vi "BBoxOne.vi"() -> ()   [LabVIEW 2021]
uses:
  D:/tmytek/Source/bbox-api/example/BBoxOne Series/LabVIEW/BBoxAPI.dll
  BBoxAPI.dll
  kernel32.dll
panel:
  out "Exists Table Filenames":string[](array[string])
  out "Get Current Working Directory":path
  in  "Set Current Working Directory":path
  in  "Target AAkit Index":u32
  in  "Target Freq Index":u32
  out "RX Board4 elementDR":dbl
  out "TX Board4  elementDR":dbl
  out "RX Board3 elementDR":dbl
  out "TX Board3 elementDR":dbl
  out "RX Board2 elementDR":dbl
  out "TX Board2 elementDR":dbl
  out "RX Board1 elementDR":dbl
  out "TX Board1 elementDR":dbl
  out "setAllChannelGain":i32
  in  "Board Number:\nRange from 1 to 4":i32=1
  in  "Board_Ch4":dbl
  in  "Board_Ch3":dbl
  in  "Board_Ch2":dbl
  in  "Board_Ch1":dbl
  out "readChannelSwitchValues":i32[][](array[numeric])
  out "Target Frequency":string
  out "Target AAKit Name":string
  out "getAAKitList":string[](array[string])
  out "RX Maximum Gain":dbl
  out "TX Maximum Gain":dbl
  out "setBeamAngle":i32(ring)=13 items=["OK"=0, "WARNING"=1, "ERROR"=2, "NO_RESPONSE"=3, "ERROR_GET_SN"=10, "ERROR_DEV_TYPE"=11, "ERROR_INIT_OBJECT"=12, "ERROR_DEV_NOT_INIT"=13, "ERROR_METHOD_NOT_FOUND"=14, "ERROR_REFLECTION"=15, "ERROR_POWER"=16, "ERROR_NETWORK_NOT_INIT"=20, "ERROR_NETWORK_INIT"=21, "ERROR_NETWORK_CONNECT_TIMEOUT"=22, "ERROR_DISCONNECT"=23, "ERROR_SOCKET"=24, "ERROR_SEND_CMD"=25, "ERROR_RESP_CMD"=26, "ERROR_DEV_COUNT_ZERO"=30, "ERROR_CMD"=40, "ERROR_CMD_INIT"=41, "ERROR_BF_AAKIT"=100, "ERROR_BF_NO_AAKIT"=101, "ERROR_BF_CALI_PATH"=102, "ERROR_BF_BEAMXY"=103, "ERROR_BF_GEN"=104, "ERROR_BF_TRMODE"=105, "STATUS_BF_LOAD_CALI_INCOMPLTE"=106, "ERROR_BF_LOAD_CALI_PARSE_FAILED"=107, "ERROR_FREQ_EQUATION"=250, "ERROR_PLO_CRC"=251, "WARNING_HARMONIC"=252, "ERROR_HARMONIC_BLOCK"=253]
  in  "Phi:\nRange from 0 to 359":i32=30 min=-45 max=45 step=1
  out "switchChannelPower":string
  in  "Power :\nON = 0 OFF = 1":i32
  out "selectAAKit":i32(ring) items=["OK"=0, "WARNING"=1, "ERROR"=2, "NO_RESPONSE"=3, "ERROR_GET_SN"=10, "ERROR_DEV_TYPE"=11, "ERROR_INIT_OBJECT"=12, "ERROR_DEV_NOT_INIT"=13, "ERROR_METHOD_NOT_FOUND"=14, "ERROR_REFLECTION"=15, "ERROR_POWER"=16, "ERROR_NETWORK_NOT_INIT"=20, "ERROR_NETWORK_INIT"=21, "ERROR_NETWORK_CONNECT_TIMEOUT"=22, "ERROR_DISCONNECT"=23, "ERROR_SOCKET"=24, "ERROR_SEND_CMD"=25, "ERROR_RESP_CMD"=26, "ERROR_DEV_COUNT_ZERO"=30, "ERROR_CMD"=40, "ERROR_CMD_INIT"=41, "ERROR_BF_AAKIT"=100, "ERROR_BF_NO_AAKIT"=101, "ERROR_BF_CALI_PATH"=102, "ERROR_BF_BEAMXY"=103, "ERROR_BF_GEN"=104, "ERROR_BF_TRMODE"=105, "STATUS_BF_LOAD_CALI_INCOMPLTE"=106, "ERROR_BF_LOAD_CALI_PARSE_FAILED"=107, "ERROR_FREQ_EQUATION"=250, "ERROR_PLO_CRC"=251, "WARNING_HARMONIC"=252, "ERROR_HARMONIC_BLOCK"=253]
  out "readBeamPhaseValues":i32[][](array[numeric])
  out "readBeamGainValues":dbl[][](array[numeric])
  in  "Theta:\nRange from 0 to 45":i32=15 min=-45 max=45 step=1
  in  "Beam Gain:\nIn tx_mode : \ntx_min_gain to tx_max_gain\nIn rx mode : \nrx_min_gain to to rx_max_gain":dbl=1.0 step=0.5
  out "setChannelGainPhase":string
  in  "deg range from 0 to 355":i32 min=0 max=355 step=5
  in  "db range:\nIn tx_mode : \ntx_min_gain to tx_max_gain\nIn rx mode : \nrx_min_gain to to rx_max_gain":dbl step=0.5
  in  "Channel:\n Range from 1 to 16":i32=16 min=1 max=16
  in  "Mode : \nTX = 1 \nRX = 2":i32=1 min=1 max=2 step=1
  out "RX Minimum Gain":dbl
  out "TX Minimum Gain":dbl
  out "Current Mode":i32
  out "SwitchTxRxMode":i32(ring) items=["OK"=0, "WARNING"=1, "ERROR"=2, "NO_RESPONSE"=3, "ERROR_GET_SN"=10, "ERROR_DEV_TYPE"=11, "ERROR_INIT_OBJECT"=12, "ERROR_DEV_NOT_INIT"=13, "ERROR_METHOD_NOT_FOUND"=14, "ERROR_REFLECTION"=15, "ERROR_POWER"=16, "ERROR_NETWORK_NOT_INIT"=20, "ERROR_NETWORK_INIT"=21, "ERROR_NETWORK_CONNECT_TIMEOUT"=22, "ERROR_DISCONNECT"=23, "ERROR_SOCKET"=24, "ERROR_SEND_CMD"=25, "ERROR_RESP_CMD"=26, "ERROR_DEV_COUNT_ZERO"=30, "ERROR_CMD"=40, "ERROR_CMD_INIT"=41, "ERROR_BF_AAKIT"=100, "ERROR_BF_NO_AAKIT"=101, "ERROR_BF_CALI_PATH"=102, "ERROR_BF_BEAMXY"=103, "ERROR_BF_GEN"=104, "ERROR_BF_TRMODE"=105, "STATUS_BF_LOAD_CALI_INCOMPLTE"=106, "ERROR_BF_LOAD_CALI_PARSE_FAILED"=107, "ERROR_FREQ_EQUATION"=250, "ERROR_PLO_CRC"=251, "WARNING_HARMONIC"=252, "ERROR_HARMONIC_BLOCK"=253]
  out "setOperatingFreq":i32(ring)=13 items=["OK"=0, "WARNING"=1, "ERROR"=2, "NO_RESPONSE"=3, "ERROR_GET_SN"=10, "ERROR_DEV_TYPE"=11, "ERROR_INIT_OBJECT"=12, "ERROR_DEV_NOT_INIT"=13, "ERROR_METHOD_NOT_FOUND"=14, "ERROR_REFLECTION"=15, "ERROR_POWER"=16, "ERROR_NETWORK_NOT_INIT"=20, "ERROR_NETWORK_INIT"=21, "ERROR_NETWORK_CONNECT_TIMEOUT"=22, "ERROR_DISCONNECT"=23, "ERROR_SOCKET"=24, "ERROR_SEND_CMD"=25, "ERROR_RESP_CMD"=26, "ERROR_DEV_COUNT_ZERO"=30, "ERROR_CMD"=40, "ERROR_CMD_INIT"=41, "ERROR_BF_AAKIT"=100, "ERROR_BF_NO_AAKIT"=101, "ERROR_BF_CALI_PATH"=102, "ERROR_BF_BEAMXY"=103, "ERROR_BF_GEN"=104, "ERROR_BF_TRMODE"=105, "STATUS_BF_LOAD_CALI_INCOMPLTE"=106, "ERROR_BF_LOAD_CALI_PARSE_FAILED"=107, "ERROR_FREQ_EQUATION"=250, "ERROR_PLO_CRC"=251, "WARNING_HARMONIC"=252, "ERROR_HARMONIC_BLOCK"=253]
  out "getFrequencyList":string[](array[string])
  out "Init":i32(ring)=13 items=["OK"=0, "WARNING"=1, "ERROR"=2, "NO_RESPONSE"=3, "ERROR_GET_SN"=10, "ERROR_DEV_TYPE"=11, "ERROR_INIT_OBJECT"=12, "ERROR_DEV_NOT_INIT"=13, "ERROR_METHOD_NOT_FOUND"=14, "ERROR_REFLECTION"=15, "ERROR_POWER"=16, "ERROR_NETWORK_NOT_INIT"=20, "ERROR_NETWORK_INIT"=21, "ERROR_NETWORK_CONNECT_TIMEOUT"=22, "ERROR_DISCONNECT"=23, "ERROR_SOCKET"=24, "ERROR_SEND_CMD"=25, "ERROR_RESP_CMD"=26, "ERROR_DEV_COUNT_ZERO"=30, "ERROR_CMD"=40, "ERROR_CMD_INIT"=41, "ERROR_BF_AAKIT"=100, "ERROR_BF_NO_AAKIT"=101, "ERROR_BF_CALI_PATH"=102, "ERROR_BF_BEAMXY"=103, "ERROR_BF_GEN"=104, "ERROR_BF_TRMODE"=105, "STATUS_BF_LOAD_CALI_INCOMPLTE"=106, "ERROR_BF_LOAD_CALI_PARSE_FAILED"=107, "ERROR_FREQ_EQUATION"=250, "ERROR_PLO_CRC"=251, "WARNING_HARMONIC"=252, "ERROR_HARMONIC_BLOCK"=253]
  out "SN":string
  out "ScanningDevice":string[](array[string])
  # "Notice:\n\nThe Set / Get Current Working Diectory Path must be \nthe sample code directory path\n\nbbox-api\\example\\BBoxOne Series\\LabVIEW\\\n\nand must exist\n\nbbox-api\\example\\BBoxOne Series\\LabVIEW\\BBoxAPI.dll\n\nbbox-api\\example\\BBoxOne Series\\LabVIEW\\files\\\n\nbbox-api\\example\\BBoxOne Series\\LabVIEW\\logs\\\n\n---\n\n1. setChannelGainPhase(int board, int ch, double db, int deg,string sn)\n \n  The formula of channel number(1 ~ 16) to board (1 ~ 4) and ch (1 ~ 4) :\n\n   (1) board = ((channel number - 1) / 4) + 1\n   (2) ch = ((channel number - 1) % 4) +1\n\n---\n\n2. setAllChannelGain(int board, double ch1_db,double ch2_db,double ch3_db, double ch4_db, string sn)\n\n  The channel gain settings on the same board should not exceed the board elementDR. \n\n   (1) board = ((channel number - 1) / 4) + 1\n   (2) Example\n           - board = 1\n           - TX DR = (-5.5 db to 10.5 db) \n           - TX elementDR =   4.5 db\n\n            - Valid Settings :\n               ch1_db = 10.5 db\n               ch2_db = 6 db\n               ch3_db = 10 db\n               ch4_db = 8 db  \n\n\n            - Invalid Settings (ch1_db and ch2_db exceed 4.5 db):\n               ch1_db = 10.5 db\n               ch2_db = 5.5 db\n               ch3_db = 10 db\n               ch4_db = 8 db  \n\n---\n\n3. Channel order on GUI  in labview and TMXLab Kits s different.\n\n\n(1) TMXLAB Kits GUI Channel Order\n\nCh04  Ch03  Ch02  Ch01\n\nCh08  Ch07  Ch06  Ch05\n\nCh12  Ch11  Ch10  Ch09\n\nCh16  Ch15  Ch14  Ch13\n\n\n\n(2) Labview GUI Channel Order\n\nCh01  Ch02  Ch03  Ch04\n\nCh05  Ch06  Ch07  Ch08\n\nCh09  Ch10  Ch11  Ch12\n\nCh13  Ch14  Ch15  Ch16"
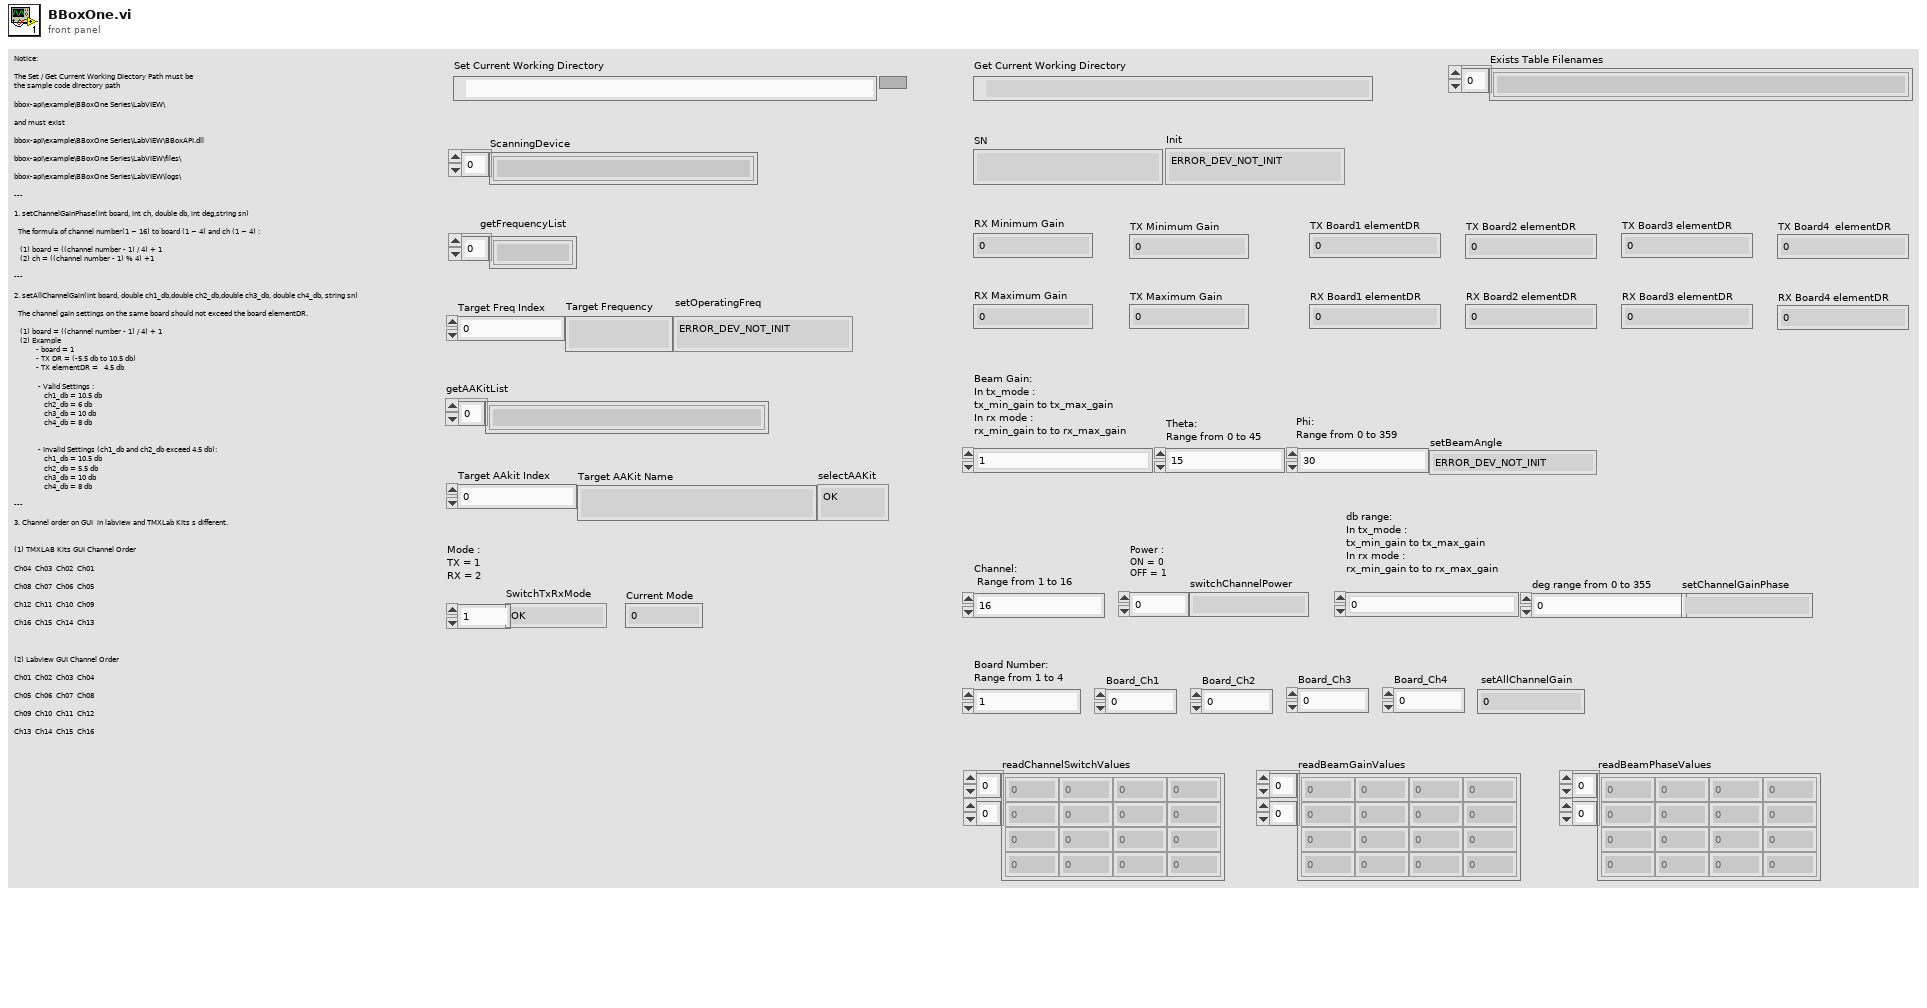
[diagram p1: front panel]
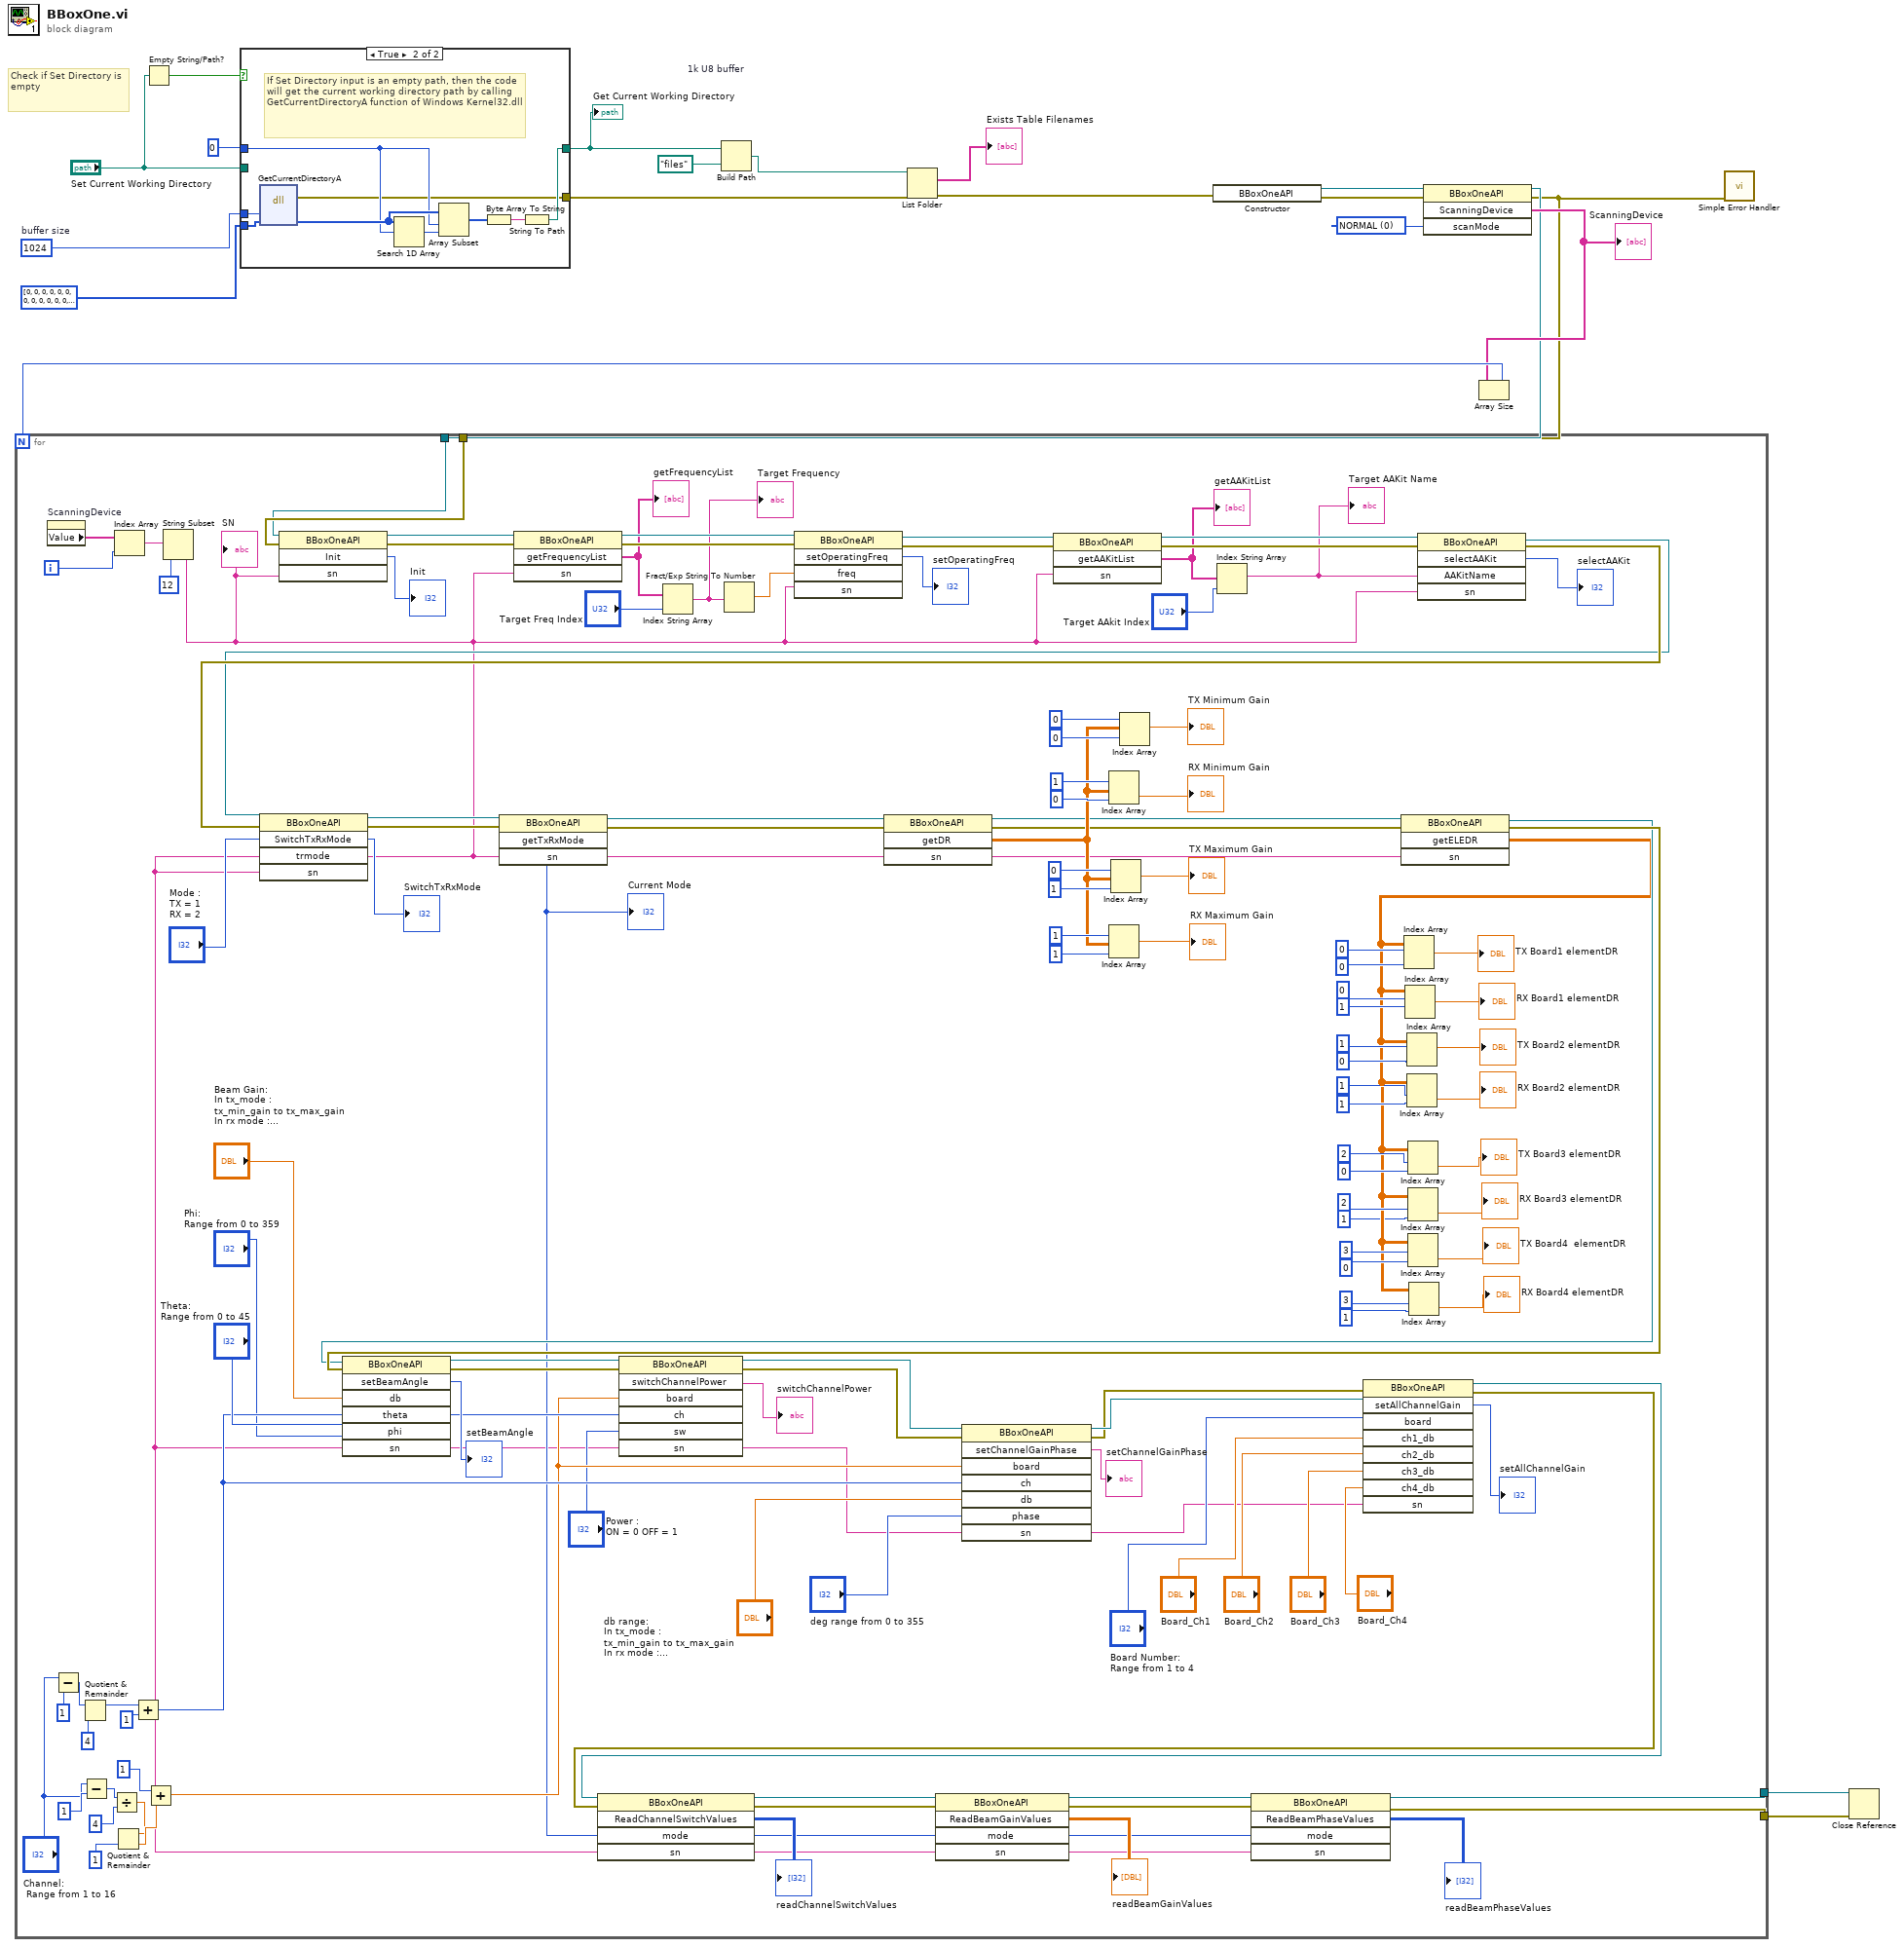
[diagram p0: block diagram]
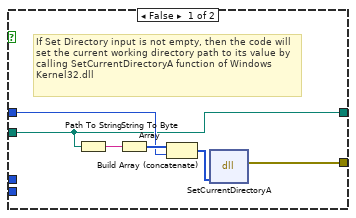
[diagram p2: hidden frame]
diagram:
  w9 = 1024  # buffer size
  w8 = u8[] [0, 0, 0, 0, 0, 0, 0, 0, 0, 0, 0, 0, 0, 0, 0, 0, 0, 0, 0, 0, 0, 0, 0, 0, 0, 0, 0, 0, 0, 0, 0, 0, 0, 0, 0, 0, 0, 0, 0, 0, 0, 0, 0, 0, 0, 0, 0, 0, 0, 0, 0, 0, 0, 0, 0, 0, 0, 0, 0, 0, 0, 0, 0, 0, 0, 0, 0, 0, 0, 0, 0, 0, 0, 0, 0, 0, 0, 0, 0, 0, 0, 0, 0, 0, 0, 0, 0, 0, 0, 0, 0, 0, 0, 0, 0, 0, 0, 0, 0, 0, 0, 0, 0, 0, 0, 0, 0, 0, 0, 0, 0, 0, 0, 0, 0, 0, 0, 0, 0, 0, 0, 0, 0, 0, 0, 0, 0, 0, 0, 0, 0, 0, 0, 0, 0, 0, 0, 0, 0, 0, 0, 0, 0, 0, 0, 0, 0, 0, 0, 0, 0, 0, 0, 0, 0, 0, 0, 0, 0, 0, 0, 0, 0, 0, 0, 0, 0, 0, 0, 0, 0, 0, 0, 0, 0, 0, 0, 0, 0, 0, 0, 0, 0, 0, 0, 0, 0, 0, 0, 0, 0, 0, 0, 0, 0, 0, 0, 0, 0, 0, 0, 0, 0, 0, 0, 0, 0, 0, 0, 0, 0, 0, 0, 0, 0, 0, 0, 0, 0, 0, 0, 0, 0, 0, 0, 0, 0, 0, 0, 0, 0, 0, 0, 0, 0, 0, 0, 0, 0, 0, 0, 0, 0, 0, 0, 0, 0, 0, 0, 0, 0, 0, 0, 0, 0, 0, 0, 0, 0, 0, 0, 0, 0, 0, 0, 0, 0, 0, 0, 0, 0, 0, 0, 0, 0, 0, 0, 0, 0, 0, 0, 0, 0, 0, 0, 0, 0, 0, 0, 0, 0, 0, 0, 0, 0, 0, 0, 0, 0, 0, 0, 0, 0, 0, 0, 0, 0, 0, 0, 0, 0, 0, 0, 0, 0, 0, 0, 0, 0, 0, 0, 0, 0, 0, 0, 0, 0, 0, 0, 0, 0, 0, 0, 0, 0, 0, 0, 0, 0, 0, 0, 0, 0, 0, 0, 0, 0, 0, 0, 0, 0, 0, 0, 0, 0, 0, 0, 0, 0, 0, 0, 0, 0, 0, 0, 0, 0, 0, 0, 0, 0, 0, 0, 0, 0, 0, 0, 0, 0, 0, 0, 0, 0, 0, 0, 0, 0, 0, 0, 0, 0, 0, 0, 0, 0, 0, 0, 0, 0, 0, 0, 0, 0, 0, 0, 0, 0, 0, 0, 0, 0, 0, 0, 0, 0, 0, 0, 0, 0, 0, 0, 0, 0, 0, 0, 0, 0, 0, 0, 0, 0, 0, 0, 0, 0, 0, 0, 0, 0, 0, 0, 0, 0, 0, 0, 0, 0, 0, 0, 0, 0, 0, 0, 0, 0, 0, 0, 0, 0, 0, 0, 0, 0, 0, 0, 0, 0, 0, 0, 0, 0, 0, 0, 0, 0, 0, 0, 0, 0, 0, 0, 0, 0, 0, 0, 0, 0, 0, 0, 0, 0, 0, 0, 0, 0, 0, 0, 0, 0, 0, 0, 0, 0, 0, 0, 0, 0, 0, 0, 0, 0, 0, 0, 0, 0, 0, 0, 0, 0, 0, 0, 0, 0, 0, 0, 0, 0, 0, 0, 0, 0, 0, 0, 0, 0, 0, 0, 0, 0, 0, 0, 0, 0, 0, 0, 0, 0, 0, 0, 0, 0, 0, 0, 0, 0, 0, 0, 0, 0, 0, 0, 0, 0, 0, 0, 0, 0, 0, 0, 0, 0, 0, 0, 0, 0, 0, 0, 0, 0, 0, 0, 0, 0, 0, 0, 0, 0, 0, 0, 0, 0, 0, 0, 0, 0, 0, 0, 0, 0, 0, 0, 0, 0, 0, 0, 0, 0, 0, 0, 0, 0, 0, 0, 0, 0, 0, 0, 0, 0, 0, 0, 0, 0, 0, 0, 0, 0, 0, 0, 0, 0, 0, 0, 0, 0, 0, 0, 0, 0, 0, 0, 0, 0, 0, 0, 0, 0, 0, 0, 0, 0, 0, 0, 0, 0, 0, 0, 0, 0, 0, 0, 0, 0, 0, 0, 0, 0, 0, 0, 0, 0, 0, 0, 0, 0, 0, 0, 0, 0, 0, 0, 0, 0, 0, 0, 0, 0, 0, 0, 0, 0, 0, 0, 0, 0, 0, 0, 0, 0, 0, 0, 0, 0, 0, 0, 0, 0, 0, 0, 0, 0, 0, 0, 0, 0, 0, 0, 0, 0, 0, 0, 0, 0, 0, 0, 0, 0, 0, 0, 0, 0, 0, 0, 0, 0, 0, 0, 0, 0, 0, 0, 0, 0, 0, 0, 0, 0, 0, 0, 0, 0, 0, 0, 0, 0, 0, 0, 0, 0, 0, 0, 0, 0, 0, 0, 0, 0, 0, 0, 0, 0, 0, 0, 0, 0, 0, 0, 0, 0, 0, 0, 0, 0, 0, 0, 0, 0, 0, 0, 0, 0, 0, 0, 0, 0, 0, 0, 0, 0, 0, 0, 0, 0, 0, 0, 0, 0, 0, 0, 0, 0, 0, 0, 0, 0, 0, 0, 0, 0, 0, 0, 0, 0, 0, 0, 0, 0, 0, 0, 0, 0, 0, 0, 0, 0, 0, 0, 0, 0, 0, 0, 0, 0, 0, 0, 0, 0, 0, 0, 0, 0, 0, 0, 0, 0, 0, 0, 0, 0, 0, 0, 0, 0, 0, 0, 0, 0, 0, 0, 0, 0, 0, 0, 0, 0, 0, 0, 0, 0, 0, 0, 0, 0, 0, 0, 0, 0, 0, 0, 0, 0, 0, 0, 0, 0, 0, 0, 0, 0, 0, 0, 0, 0, 0, 0, 0, 0, 0, 0, 0, 0, 0, 0, 0, 0, 0, 0, 0, 0, 0, 0, 0, 0, 0, 0, 0, 0, 0, 0, 0, 0, 0, 0, 0, 0, 0, 0, 0, 0, 0, 0, 0, 0, 0, 0, 0, 0, 0, 0, 0, 0, 0, 0, 0, 0, 0, 0, 0, 0, 0, 0, 0, 0, 0, 0, 0, 0, 0, 0, 0, 0, 0, 0, 0, 0, 0, 0, 0, 0, 0, 0, 0, 0, 0, 0, 0, 0, 0, 0, 0, 0, 0, 0, 0, 0, 0, 0, 0, 0, 0, 0, 0, 0, 0, 0, 0, 0, 0, 0, 0, 0, 0, 0, 0, 0, 0, 0, 0, 0, 0, 0, 0, 0, 0]  # 1k U8 buffer
  w20 = 0 items=["NORMAL", "FAST"] ("scanMode")
  # "Check if Set Directory is empty"
  n1 = Empty String/Path?(string/path="Set Current Working Directory") -> (empty?=w10:bool)
  n2 = case shown="True" w10 {
    tunnel: "Set Current Working Directory" -> [w22 _]
    tunnel: u8 0 -> [w24 w31]
    tunnel: w9 -> [_ w30]
    tunnel: w8 -> [_ w29]
    tunnel: [w22 w28] -> w3
    tunnel: [w21 w27] -> w6
    frame False {
      # "If Set Directory input is not empty, then the code will set the current working directory path to its value by calling SetCurrentDirectoryA function of Windows Kernel32.dll"
      n3 = Path To String(path=w22) -> (string=w23:string)
      n4 = String To Byte Array(string=w23) -> (unsigned byte array=w26:u8[])
      n5 = Build Array (concatenate)(w26, w24) -> (w25:u8[])
      n6 = dll-call lib="Kernel32.dll" fn="SetCurrentDirectoryA" label="Kernel32.dll - \nSetCurrentDirectoryA"("lpPathName"=w25) -> (error out=w21:errorcluster)  [unwired: 4 in, 2 out]
    }
    frame True {
      # "If Set Directory input is an empty path, then the code will get the current working directory path by calling GetCurrentDirectoryA function of Windows Kernel32.dll"
      n7 = dll-call lib="kernel32.dll" fn="GetCurrentDirectoryA" label="Kernel32.dll - \nGetCurrentDirectoryA"("nBufferLength"=w30, "lpBuffer"=w29) -> (error out=w27:errorcluster, "lpBuffer"=w34:u8[])  [unwired: 4 in, 2 out]
      n8 = Search 1D Array(1D array=w34, element=w31) -> (index of element=w35:i32)  [unwired: 1 out]
      n9 = Array Subset(array=w34, index=w31, length=w35) -> (w32:u8[])
      n10 = Byte Array To String(unsigned byte array=w32) -> (string=w33:string)
      n11 = String To Path(string=w33) -> (path=w28:path)
    }
  }
  "Get Current Working Directory" <- w3
  n12 = Build Path(base path=w3, name or relative path=path "files") -> (appended path=w1:path)
  n13 = List Folder(path=w1, error in=w6) -> (filenames=→"Exists Table Filenames":string[], error out=w5:errorcluster)  [unwired: 2 in, 2 out]
  n14 = constructor class="BBoxOneAPI"(error in=w5) -> (reference out=w19:refnum<k24>, error out=w18:errorcluster)  [unwired: 2 in, 1 out]
  n15 = invoke class="BBoxOneAPI" method="ScanningDevice"(reference=w19, error in=w18, "scanMode"=w20) -> (reference out=w15:refnum<k24>, error out=w14:errorcluster, "ScanningDevice"=w16:string[])  [unwired: 1 in, 1 out]
  "ScanningDevice" <- w16
  n16 = Array Size(array=w16) -> (size(s)=w17:i32)
  n17 = for {
    N: w17 -> [_]
    tunnel: w15 -> [w124]
    tunnel: w14 -> [w156]
    tunnel: [w37] -> w13
    tunnel: [w36] -> w12
    i -> [w66]
    n18 = property on="ScanningDevice" class="Arr (strict)"() -> ("Value"=w134:string[])  [unwired: 2 in, 2 out]
    n19 = Subtract(x="Channel:\n Range from 1 to 16", y=1) -> (x-y=w99:i32)
    n20 = Quotient & Remainder(x=w99, y=4) -> (x-y*floor(x/y)=w97:i32)  [unwired: 1 out]
    n21 = Subtract(x="Channel:\n Range from 1 to 16", y=1) -> (x-y=w110:i32)
    n22 = Divide(x=w110, y=4) -> (x/y=w103:dbl)
    n23 = Quotient & Remainder(x=w103, y=1) -> (floor(x/y)=w106:dbl)  [unwired: 1 out]
    n24 = Index Array(array=w134, index=w66) -> (element=w158:string)
    n25 = Add(x=w97, y=1) -> (x+y=w105:i32)
    n26 = Add(x=1, y=w106) -> (x+y=w104:dbl)
    n27 = String Subset(string=w158, length (rest)=12) -> (substring=w38:string)  [unwired: 1 in]
    "SN" <- w38
    n28 = invoke class="BBoxOneAPI" method="Init"(reference=w124, error in=w156, "sn"=w38) -> (reference out=w133:refnum<k24>, error out=w132:errorcluster, "Init"=→"Init":i32)  [unwired: 1 in, 1 out]
    n29 = invoke class="BBoxOneAPI" method="getFrequencyList"(reference=w133, error in=w132, "sn"=w38) -> (reference out=w131:refnum<k24>, error out=w130:errorcluster, "getFrequencyList"=w121:string[])  [unwired: 1 in, 1 out]
    "getFrequencyList" <- w121
    n30 = Index String Array(1:"Target Freq Index", 2:w121) -> (0:w117:string)  [unwired: 1 in]
    "Target Frequency" <- w117
    n31 = Fract/Exp String To Number(string=w117) -> (number=w122:dbl)  [unwired: 3 in, 1 out]
    n32 = invoke class="BBoxOneAPI" method="setOperatingFreq"(reference=w131, error in=w130, "freq"=w122, "sn"=w38) -> (reference out=w138:refnum<k24>, error out=w137:errorcluster, "setOperatingFreq"=→"setOperatingFreq":i32)  [unwired: 1 in, 2 out]
    n33 = invoke class="BBoxOneAPI" method="getAAKitList"(reference=w138, error in=w137, "sn"=w38) -> (reference out=w136:refnum<k24>, error out=w135:errorcluster, "getAAKitList"=w119:string[])  [unwired: 1 in, 1 out]
    "getAAKitList" <- w119
    n34 = Index String Array(1:"Target AAkit Index", 2:w119) -> (0:w118:string)  [unwired: 1 in]
    "Target AAKit Name" <- w118
    n35 = invoke class="BBoxOneAPI" method="selectAAKit"(reference=w136, error in=w135, "AAKitName"=w118, "sn"=w38) -> (reference out=w123:refnum<k24>, error out=w126:errorcluster, "selectAAKit"=→"selectAAKit":i32)  [unwired: 1 in, 2 out]
    n36 = invoke class="BBoxOneAPI" method="SwitchTxRxMode"(reference=w123, error in=w126, "trmode"="Mode : \nTX = 1 \nRX = 2", "sn"=w38) -> (reference out=w153:refnum<k24>, error out=w152:errorcluster, "SwitchTxRxMode"=→"SwitchTxRxMode":i32)  [unwired: 1 in, 2 out]
    n37 = invoke class="BBoxOneAPI" method="getTxRxMode"(reference=w153, error in=w152, "sn"=w38) -> (reference out=w151:refnum<k24>, error out=w150:errorcluster, "getTxRxMode"=w39:i32)  [unwired: 1 in, 1 out]
    "Current Mode" <- w39
    n38 = invoke class="BBoxOneAPI" method="getDR"(reference=w151, error in=w150, "sn"=w38) -> (reference out=w71:refnum<k24>, error out=w70:errorcluster, "getDR"=w127:dbl[][])  [unwired: 1 in, 1 out]
    n39 = Index Array(array=w127, index (row)=1, index (col)=0) -> (element=→"RX Minimum Gain":dbl)
    n40 = Index Array(array=w127, index (row)=1, index (col)=1) -> (element=→"RX Maximum Gain":dbl)
    n41 = Index Array(array=w127, index (row)=0, index (col)=1) -> (element=→"TX Maximum Gain":dbl)
    n42 = Index Array(array=w127, index (row)=0, index (col)=0) -> (element=→"TX Minimum Gain":dbl)
    n43 = invoke class="BBoxOneAPI" method="getELEDR"(reference=w71, error in=w70, "sn"=w38) -> (reference out=w65:refnum<k24>, error out=w69:errorcluster, "getELEDR"=w42:dbl[][])  [unwired: 1 in, 1 out]
    n44 = invoke class="BBoxOneAPI" method="setBeamAngle"(reference=w65, error in=w69, "db"="Beam Gain:\nIn tx_mode : \ntx_min_gain to tx_max_gain\nIn rx mode : \nrx_min_gain to to rx_max_gain", "theta"="Theta:\nRange from 0 to 45", "phi"="Phi:\nRange from 0 to 359", "sn"=w38) -> (reference out=w90:refnum<k24>, error out=w89:errorcluster, "setBeamAngle"=→"setBeamAngle":i32)  [unwired: 1 in, 4 out]
    n45 = invoke class="BBoxOneAPI" method="switchChannelPower"(reference=w90, error in=w89, "board"=w104, "ch"=w105, "sw"="Power :\nON = 0 OFF = 1", "sn"=w38) -> (reference out=w88:refnum<k24>, error out=w87:errorcluster, "switchChannelPower"=→"switchChannelPower":string)  [unwired: 1 in, 4 out]
    n46 = invoke class="BBoxOneAPI" method="setChannelGainPhase"(reference=w88, error in=w87, "board"=w104, "ch"=w105, "db"="db range:\nIn tx_mode : \ntx_min_gain to tx_max_gain\nIn rx mode : \nrx_min_gain to to rx_max_gain", "phase"="deg range from 0 to 355", "sn"=w38) -> (reference out=w80:refnum<k24>, error out=w79:errorcluster, "setChannelGainPhase"=→"setChannelGainPhase":string)  [unwired: 1 in, 5 out]
    n47 = invoke class="BBoxOneAPI" method="setAllChannelGain"(reference=w80, error in=w79, "board"="Board Number:\nRange from 1 to 4", "ch1_db"="Board_Ch1", "ch2_db"="Board_Ch2", "ch3_db"="Board_Ch3", "ch4_db"="Board_Ch4", "sn"=w38) -> (reference out=w78:refnum<k24>, error out=w77:errorcluster, "setAllChannelGain"=→"setAllChannelGain":i32)  [unwired: 1 in, 6 out]
    n48 = invoke class="BBoxOneAPI" method="ReadChannelSwitchValues"(reference=w78, error in=w77, "mode"=w39, "sn"=w38) -> (reference out=w76:refnum<k24>, error out=w75:errorcluster, "ReadChannelSwitchValues"=→"readChannelSwitchValues":i32[][])  [unwired: 1 in, 2 out]
    n49 = invoke class="BBoxOneAPI" method="ReadBeamGainValues"(reference=w76, error in=w75, "mode"=w39, "sn"=w38) -> (reference out=w74:refnum<k24>, error out=w73:errorcluster, "ReadBeamGainValues"=→"readBeamGainValues":dbl[][])  [unwired: 1 in, 2 out]
    n50 = invoke class="BBoxOneAPI" method="ReadBeamPhaseValues"(reference=w74, error in=w73, "mode"=w39, "sn"=w38) -> (reference out=w36:refnum<k24>, error out=w37:errorcluster, "ReadBeamPhaseValues"=→"readBeamPhaseValues":i32[][])  [unwired: 1 in, 2 out]
    n51 = Index Array(array=w42, index (row)=0, index (col)=0) -> (element=→"TX Board1 elementDR":dbl)
    n52 = Index Array(array=w42, index (row)=0, index (col)=1) -> (element=→"RX Board1 elementDR":dbl)
    n53 = Index Array(array=w42, index (row)=1, index (col)=0) -> (element=→"TX Board2 elementDR":dbl)
    n54 = Index Array(array=w42, index (row)=1, index (col)=1) -> (element=→"RX Board2 elementDR":dbl)
    n55 = Index Array(array=w42, index (row)=2, index (col)=0) -> (element=→"TX Board3 elementDR":dbl)
    n56 = Index Array(array=w42, index (row)=2, index (col)=1) -> (element=→"RX Board3 elementDR":dbl)
    n57 = Index Array(array=w42, index (row)=3, index (col)=0) -> (element=→"TX Board4  elementDR":dbl)
    n58 = Index Array(array=w42, index (row)=3, index (col)=1) -> (element=→"RX Board4 elementDR":dbl)
  }
  n59 = call <vilib>:"Simple Error Handler.vi"("error in (no error)"=w14) -> ()  [unwired: 4 in, 5 out]
  n60 = Close Reference(reference=w12, error in (no error)=w13) -> ()  [unwired: 1 out]
